vi "ziModSetValueDouble.vi"(8 "Error In":errorcluster, 9 "Value":dbl, 10 "Path":string="sweep/start", 11 "ModHandle In":T1 {"ModHandle" format="0x%08x"; "Conn" format="0x%08x"}) -> (0 "Error Out":errorcluster, 3 "ModHandle Out":T1 {"ModHandle" format="0x%08x"; "Conn" format="0x%08x"})   [LabVIEW 2018, in "Zurich Instruments LabOne.lvlib"]
doc: "This vi sets values of the specified <b>module </b> nodes in <b>Path</b> to <b>Value</b>., e.g sweep/endless."
uses:
  Zurich Instruments LabOne.lvlib
  <instrlib>/Zurich Instruments LabOne/Private/ziLV64.framework
  ziTypeModHandle.ctl
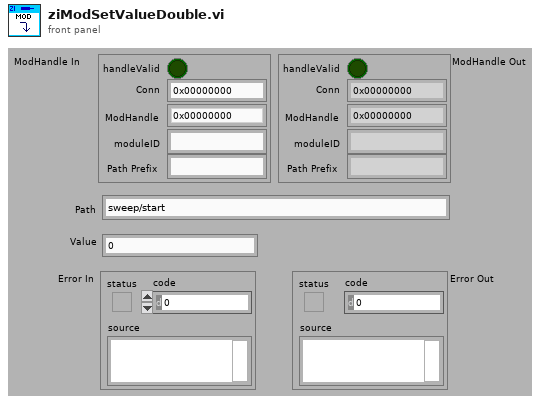
[diagram p1: front panel]
types:
  T1 = typedef "Zurich Instruments LabOne.lvlib/ziTypeModHandle.ctl" = cluster{"handleValid":bool, "Conn":u64, "ModHandle":u64, "moduleID":string, "Path Prefix":string}
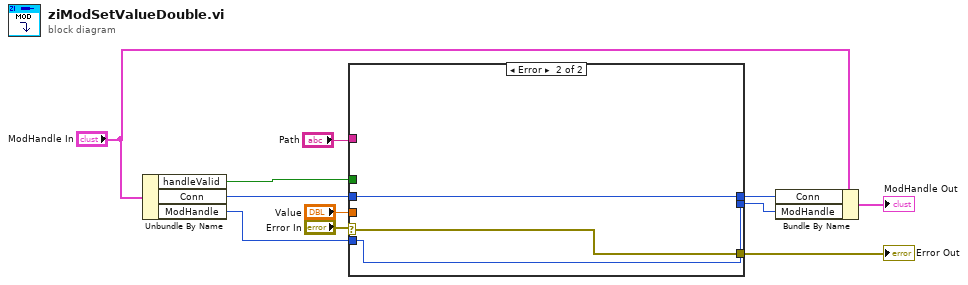
[diagram p0: block diagram]
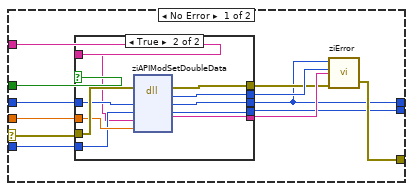
[diagram p2: hidden frame]
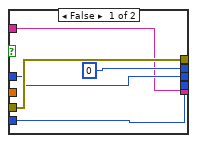
[diagram p3: hidden frame]
diagram:
  n1 = Unbundle By Name("ModHandle In") -> ("handleValid"=w3:bool, "Conn"=w4:u64, "ModHandle"=w6:u64)
  n2 = case shown="Error" "Error In" {
    selector: "Error In" -> [w19 w41]
    tunnel: "Value" -> [w23 _]
    tunnel: [w22 w41] -> w1
    tunnel: "Path" -> [w15 _]
    tunnel: w6 -> [w18 w40]
    tunnel: [w17 w40] -> w5
    tunnel: [w12 w39] -> w2
    tunnel: w4 -> [w16 w39]
    tunnel: w3 -> [w14 _]
    frame No Error {
      n3 = case shown="True" w14 {
        tunnel: w19 -> [w28 w38]
        tunnel: w23 -> [_ w37]
        tunnel: [w28 w36] -> w13
        tunnel: [u32 0 ("return type") w35] -> w21
        tunnel: [w25 w34] -> w12
        tunnel: [w24 w33] -> w20
        tunnel: w18 -> [w26 w32]
        tunnel: [w26 w31] -> w17
        tunnel: w16 -> [w25 w30]
        tunnel: w15 -> [w24 w29]
        frame False {
        }
        frame True {
          n4 = dll-call lib="Applications/National Instruments/LabVIEW 2019 64-bit/instr.lib/Zurich Instruments LabOne/Private/ziLV*.*" fn="ziAPIModSetDoubleData"(error in=w38, "Conn"=w30, "ModHandle"=w32, "Path"=w29, "Value"=w37) -> (error out=w36:errorcluster, "return type"=w35:u32, "Conn"=w34:u64, "ModHandle"=w31:u64, "Path"=w33:string)  [unwired: 3 in, 1 out]
        }
      }
      n5 = call "ziError.vi"("Conn"=w12, "ziErrorCode"=w21, "Error In"=w13, "Annotation"=w20) -> ("Error Out"=w22:errorcluster)  [unwired: 1 in, 1 out]
    }
    frame Error {
    }
  }
  "Error Out" <- w1
  n6 = Bundle By Name(cluster="ModHandle In", "Conn"=w2, "ModHandle"=w5) -> (→"ModHandle Out":T1)
